vi "Extract Header and Set Position File.vi"(8 "error IO":errorcluster, 11 "Binary File":path) -> (0 "error out":errorcluster, 1 "refnum out":refnum<file>, 2 "Height":u32, 3 "Width":u32, 4 "Image/Sector Size(bytes)":i64, 5 "Mask ROI Out":T1={"left annulus"={"Center X"=929, "Center Y"=663, "Inner Radius"=200, "Outer Radius"=405, "Start Angle"=90.0, "End Angle"=180.0}, "right annulus"={"Center X"=929, "Center Y"=663, "Inner Radius"=200, "Outer Radius"=405, "Start Angle"=90.0, "End Angle"=180.0}, "Threshold Range"={"Lower value"=106.82432432432432, "Upper value"=255.0}, "[Avg BG]"=[0, 0, 0, 0, 0, 0, 0, 0, 0, 0, 0, 0, 0, 0, 0, 0, 0, 0, 0, 0, 0, 0, 0, 0, 0, 0, 0, 0, 0, 0, 0, 0], "Number of Sectors"=0, "Left ROI"={"Global Rectangle"=[], "Contours"=[]}, "Right ROI"={"Global Rectangle"=[], "Contours"=[]}, "Left Start Angle Duty Cycle"=0.0, "Left End Angle Duty Cycle"=0.0, "Right End Angle Duty Cycle"=0.0, "Right Start Angle Duty Cycle"=0.0, "[Sector ROIs]"=[], "Consecutive Sector Threshold"=0} {"[Sector ROIs]"."Contours"."Type" items=["No Selection", "Point", "Line", "Rectangle", "Oval", "Polygon", "Freehand Region", "Annulus", "Unused2", "Unused3", "Broken Line", "Freehand Line", "Rotated Rectangle"]; "Right ROI"."Contours"."Type" items=["No Selection", "Point", "Line", "Rectangle", "Oval", "Polygon", "Freehand Region", "Annulus", "Unused2", "Unused3", "Broken Line", "Freehand Line", "Rotated Rectangle"]; "Left ROI"."Contours"."Type" items=["No Selection", "Point", "Line", "Rectangle", "Oval", "Polygon", "Freehand Region", "Annulus", "Unused2", "Unused3", "Broken Line", "Freehand Line", "Rotated Rectangle"]; "Threshold Range"."Upper value" min=0.0 max=255.0 scale=0.0..255.0; "Threshold Range"."Lower value" min=0.0 max=255.0 scale=0.0..255.0; "right annulus"."End Angle" format="%.2f"; "right annulus"."Start Angle" format="%.2f"; "right annulus"."Center X" scale=0.0..1024.0; "left annulus"."End Angle" format="%.2f"; "left annulus"."Start Angle" format="%.2f"; "left annulus"."Center X" scale=0.0..1024.0}, 6 "Header Size":i32)   [LabVIEW 2013]
uses:
  Image Processing/Mask ROI Cluster.ctl
  File IO/Convert Mask to Bytes Enum.ctl
panel:
  out "# of bytes for mask":u16
  out "File Size":i64
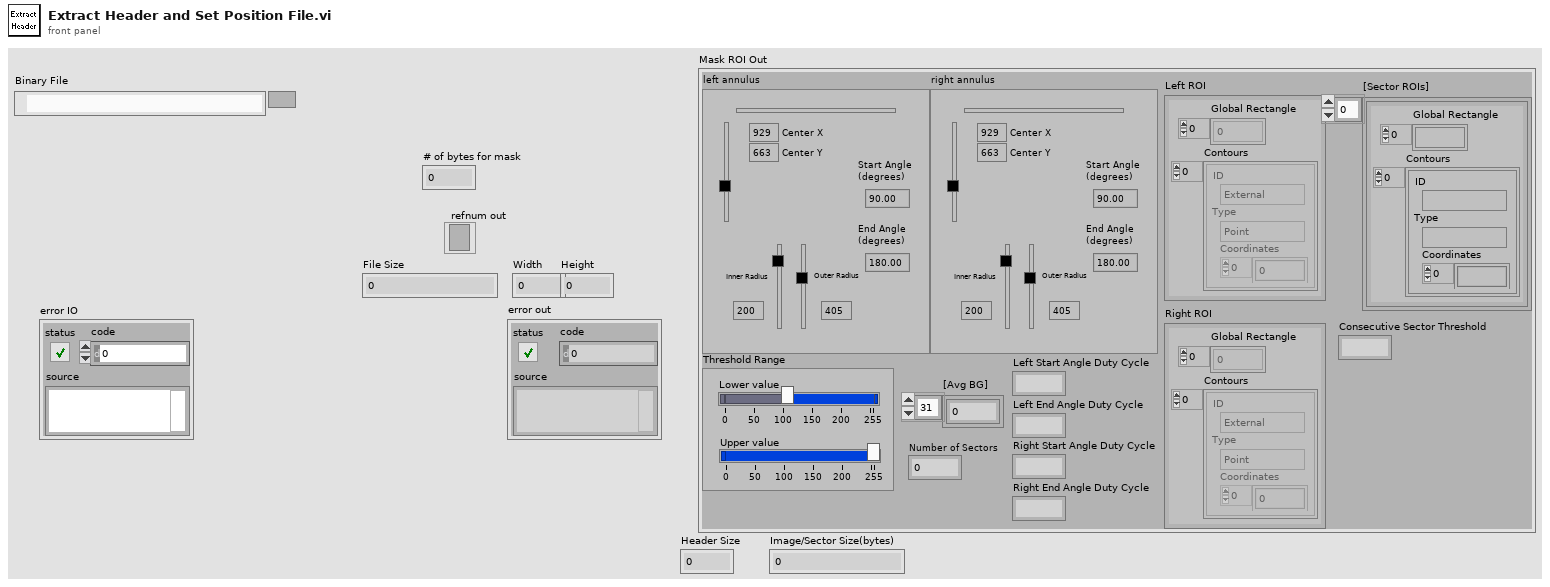
[diagram p1: front panel]
types:
  T1 = typedef "Mask ROI Cluster.ctl" = cluster{"left annulus":T2, "right annulus":T2, "Threshold Range":cluster{"Lower value":dbl, "Upper value":dbl}, "[Avg BG]":u8[], "Number of Sectors":u8, "Left ROI":T3, "Right ROI":T3, "Left Start Angle Duty Cycle":fxp<+,8,0>, "Left End Angle Duty Cycle":fxp<+,8,0>, "Right End Angle Duty Cycle":fxp<+,8,0>, "Right Start Angle Duty Cycle":fxp<+,8,0>, "[Sector ROIs]":T3[], "Consecutive Sector Threshold":u8}
  T2 = typedef "IMAQ Circle" = cluster{"Center X":i32, "Center Y":i32, "Inner Radius":i32, "Outer Radius":i32, "Start Angle":dbl, "End Angle":dbl}
  T3 = typedef "ROI Descriptor" = cluster{"Global Rectangle":i32[], "Contours":cluster{"ID":enum32{"External", "Internal"}, "Type":u32, "Coordinates":i32[]}[]}
  T4 = typedef "Convert Mask to Bytes Enum.ctl" = enum16{"Mask to Bytes", "Bytes to Mask"}
  T5 = enum16{"open", "replace", "create", "open or create", "replace or create", "replace or create with confirmation"}
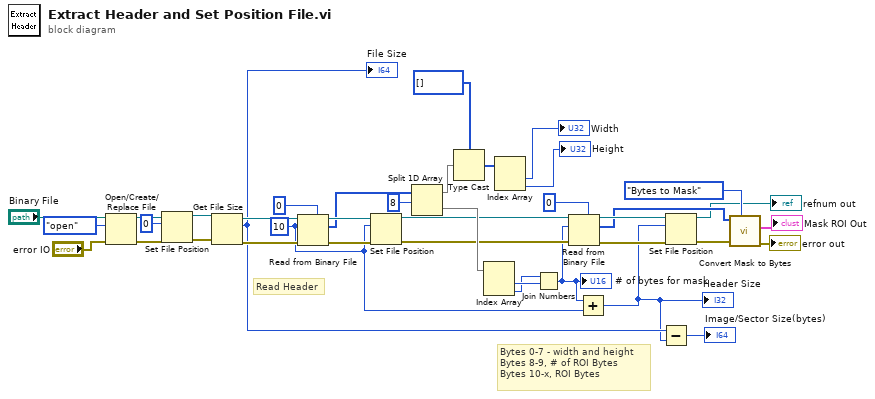
[diagram p0: block diagram]
diagram:
  w16 = 10 ("count (1)")
  # "Bytes 0-7 - width and height\nBytes 8-9, # of ROI Bytes\nBytes 10-x, ROI Bytes"
  # "Read Header"
  n1 = Open/Create/Replace File(file path (use dialog)="Binary File", error in="error IO", operation (0:open)=T5."open") -> (refnum out=w2:refnum<file>, error out=w5:errorcluster)  [unwired: 3 in, 1 out]
  n2 = Set File Position(offset (in bytes) (0)=i64 0, refnum=w2, error in=w5) -> (refnum out=w3:refnum<file>, error out=w4:errorcluster)  [unwired: 1 in]
  n3 = Get File Size(file=w3, error in=w4) -> (refnum out=w37:refnum<file>, size (in bytes)=w9:i64, 0:w38:errorcluster)
  "File Size" <- w9
  n4 = Read from Binary File(5:u8 0, 8:w38, 10:w16, 11:w37) -> (0:w30:errorcluster, 2:w28:u8[], 3:w31:refnum<file>)  [unwired: 2 in, 1 out]
  n5 = Set File Position(offset (in bytes) (0)=w16, refnum=w31, error in=w30) -> (refnum out=w21:refnum<file>, error out=w22:errorcluster)  [unwired: 1 in]
  n6 = Split 1D Array(array=w28, index=8) -> (first subarray=w26:u8[], second subarray=w25:u8[])
  n7 = Type Cast(type=u32[] [], x=w26) -> (*(type *) &x=w29:u32[])
  n8 = Index Array(array=w25) -> (element #1=w24:u8, element #2=w23:u8)  [unwired: 2 in]
  n9 = Index Array(array=w29) -> (element #1=→"Width":u32, element #2=→"Height":u32)  [unwired: 2 in]
  n10 = Join Numbers(hi=w23, lo=w24) -> ((hi.lo)=w17:u16)
  "# of bytes for mask" <- w17
  n11 = Read from Binary File(5:u8 0, 8:w22, 10:w17, 11:w21) -> (0:w19:errorcluster, 2:w14:u8[], 3:w18:refnum<file>)  [unwired: 2 in, 1 out]
  n12 = Add(x=w17, y=w16) -> (x+y=w8:i32)
  "Header Size" <- w8
  n13 = Subtract(x=w9, y=w8) -> (x-y=→"Image/Sector Size(bytes)":i64)
  n14 = Set File Position(offset (in bytes) (0)=w8, refnum=w18, error in=w19) -> (refnum out=→"refnum out":refnum<file>, error out=w15:errorcluster)  [unwired: 1 in]
  n15 = call "Convert Mask to Bytes.vi"("Mode"=Convert_Mask_to_Bytes_Enum."Bytes to Mask", "error in (no error)"=w15, "Mask Bytes In"=w14) -> ("error out"=→"error out":errorcluster, "Mask ROI Out"=→"Mask ROI Out":T1)  [unwired: 6 in, 1 out]
